vi "Joystick_XBox.vi"(11 "JoystickDevRef":T2) -> (1 "Generic_Axes":dbl[](array[numeric]), 2 "Generic_Buttons":bool[](array[boolean]), 3 "Joystick_XBox":T1, 4 "POVs":i16[](array[numeric]))   [LabVIEW 2017]
uses:
  <vilib>/Rock Robotics/WPI/Joystick/WPI_JoystickDevRef.ctl
  <vilib>/Rock Robotics/WPI/Joystick/WPI_JoystickDeviceEnum.ctl
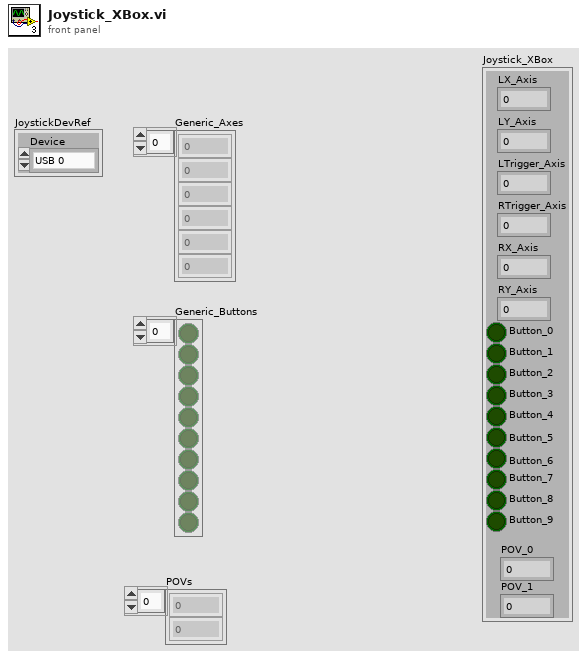
[diagram p1: front panel]
types:
  T1 = cluster{"LX_Axis":dbl, "LY_Axis":dbl, "LTrigger_Axis":dbl, "RTrigger_Axis":dbl, "RX_Axis":dbl, "RY_Axis":dbl, "Button_0":bool, "Button_1":bool, "Button_2":bool, "Button_3":bool, "Button_4":bool, "Button_5":bool, "Button_6":bool, "Button_7":bool, "Button_8":bool, "Button_9":bool, "POV_0":i16, "POV_1":i16}
  T2 = typedef "WPI_JoystickDevRef.ctl" = cluster{"Device":T3}
  T3 = typedef "WPI_JoystickDeviceEnum.ctl" = enum16{"USB 0", "USB 1", "USB 2", "USB 3", "USB 4", "USB 5"}
  T4 = cluster{"upper limit":dbl, "upper limit":dbl, "upper limit":dbl, "upper limit":dbl, "upper limit":dbl, "upper limit":dbl, bool, bool, bool, bool, bool, bool, bool, bool, bool, bool, i16, i16}
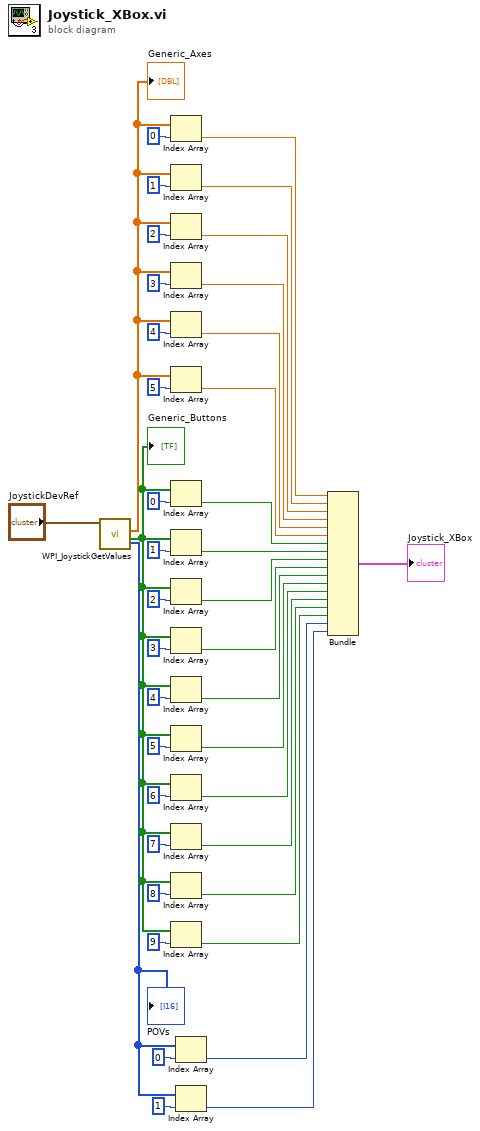
[diagram p0: block diagram]
diagram:
  n1 = call <vilib>:"WPI_JoystickGetValues.vi"("JoystickDevRef"="JoystickDevRef") -> ("Buttons"=w31:bool[], "Axes"=w24:dbl[], "POVs"=w4:i16[])  [unwired: 6 in, 2 out]
  "Generic_Axes" <- w24
  "Generic_Buttons" <- w31
  "POVs" <- w4
  n2 = Index Array(array=w24, index=0) -> (element=w23:dbl)
  n3 = Index Array(array=w24, index=1) -> (element=w22:dbl)
  n4 = Index Array(array=w24, index=2) -> (element=w21:dbl)
  n5 = Index Array(array=w24, index=3) -> (element=w20:dbl)
  n6 = Index Array(array=w24, index=4) -> (element=w19:dbl)
  n7 = Index Array(array=w24, index=5) -> (element=w18:dbl)
  n8 = Index Array(array=w31, index=0) -> (element=w17:bool)
  n9 = Index Array(array=w31, index=1) -> (element=w16:bool)
  n10 = Index Array(array=w31, index=2) -> (element=w15:bool)
  n11 = Index Array(array=w31, index=3) -> (element=w14:bool)
  n12 = Index Array(array=w31, index=4) -> (element=w13:bool)
  n13 = Index Array(array=w31, index=5) -> (element=w12:bool)
  n14 = Index Array(array=w31, index=6) -> (element=w11:bool)
  n15 = Index Array(array=w31, index=7) -> (element=w10:bool)
  n16 = Index Array(array=w31, index=8) -> (element=w9:bool)
  n17 = Index Array(array=w31, index=9) -> (element=w8:bool)
  n18 = Index Array(array=w4, index=0) -> (element=w3:i16)
  n19 = Index Array(array=w4, index=1) -> (element=w2:i16)
  n20 = Bundle("upper limit"=w23, "upper limit"=w22, "upper limit"=w21, "upper limit"=w20, "upper limit"=w19, "upper limit"=w18, w17, w16, w15, w14, w13, w12, w11, w10, w9, w8, w3, w2) -> (→"Joystick_XBox":T4)  [unwired: 1 in]
